vi "Get Edit Test Node List.vi"(8 "error in (no error)":errorcluster, 11 "Abstract Edit Test Node List Msg in":refnum<class "Abstract Edit Test Node List Msg.lvclass">) -> (0 "error out":errorcluster, 2 "Edit Test Node List":string[](array[string]), 3 "Abstract Edit Test Node List Msg out":refnum<class "Abstract Edit Test Node List Msg.lvclass">)   [LabVIEW 2013, in "Edit Test Node Model.lvlib" / "Abstract Edit Test Node List Msg.lvclass"]
uses:
  Abstract Edit Test Node List Msg.lvclass
  Abstract Edit Test Node List Msg.lvclass/Abstract Edit Test Node List Msg.ctl
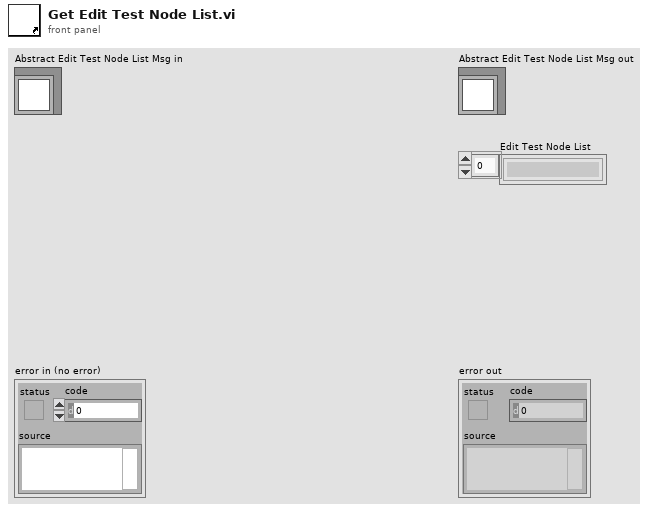
[diagram p1: front panel]
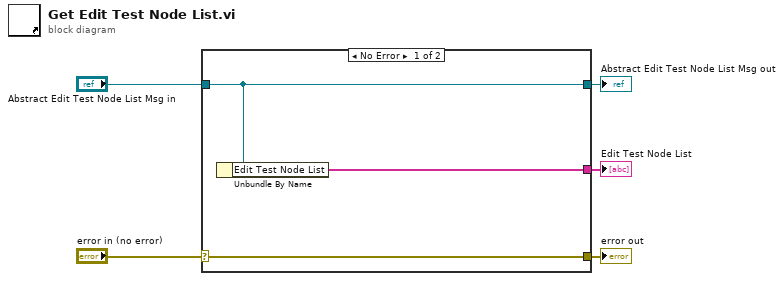
[diagram p0: block diagram]
diagram:
  n1 = case shown="No Error" "error in (no error)" {
    selector: "error in (no error)" -> [w8 w9]
    tunnel: [w8 w9] -> w4
    tunnel: [w7 w10] -> w2
    tunnel: "Abstract Edit Test Node List Msg in" -> [w7 w10]
    tunnel: [w6 _] -> w1
    frame No Error {
      n2 = Unbundle By Name(w7) -> ("Edit Test Node List"=w6:string[])
    }
    frame Error {
    }
  }
  "error out" <- w4
  "Abstract Edit Test Node List Msg out" <- w2
  "Edit Test Node List" <- w1
